vi "Tag initialize.vi"() -> (14 "RMS tag":refnum<class "NI Skyline Tag.lvclass">, 15 "RPM tag":refnum<class "NI Skyline Tag.lvclass">, 16 "Voltage tag":refnum<class "NI Skyline Tag.lvclass">, 17 "Current Tag":refnum<class "NI Skyline Tag.lvclass">, 18 "Temper tag":refnum<class "NI Skyline Tag.lvclass">, 19 "error out":errorcluster)   [LabVIEW 2017]
uses:
  <vilib>/Skyline/Tag/Wrapper/Wrapper_class/NI Skyline Tag.lvclass
  <vilib>/Skyline/Tag/Shared/typedefs/DataType.ctl
  <vilib>/Skyline/Tag/Wrapper/Wrapper AMQP_class/Open Tag AMQP.vi
  <vilib>/Skyline/Tag/Wrapper/Wrapper AMQP_class/NI Skyline Tag AMQP.lvclass
  <vilib>/Skyline/Tag/Shared/NI Skyline Tag.lvlib
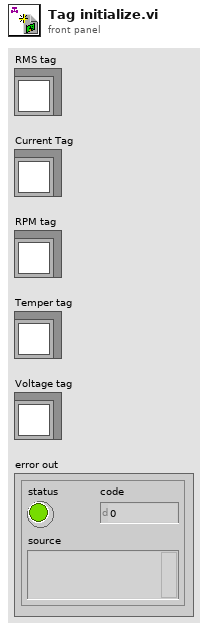
[diagram p1: front panel]
types:
  T1 = typedef "NI Skyline Tag.lvlib/DataType.ctl" = enum32{"Double", "I32", "String", "Boolean", "U64", "Timestamp"}
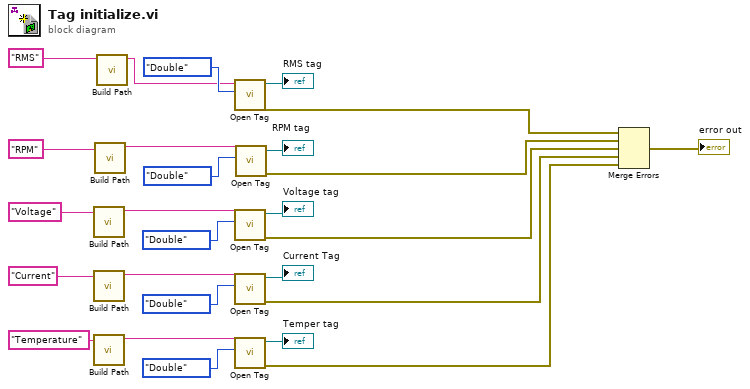
[diagram p0: block diagram]
diagram:
  n1 = call <vilib>:"Build Path.vi"("tag name"="Voltage" ("tag path")) -> ("path"=w9:string)  [unwired: 10 in]
  n2 = call <vilib>:"Build Path.vi"("tag name"="Current" ("tag path")) -> ("path"=w14:string)  [unwired: 10 in]
  n3 = call <vilib>:"Build Path.vi"("tag name"="Temperature" ("tag path")) -> ("path"=w15:string)  [unwired: 10 in]
  n4 = call <vilib>:"Build Path.vi"("tag name"="RPM" ("tag path")) -> ("path"=w7:string)  [unwired: 10 in]
  n5 = call <vilib>:"Build Path.vi"("tag name"="RMS" ("tag path")) -> ("path"=w5:string)  [unwired: 10 in]
  n6 = call-poly <vilib>:"Open Tag.vi"("data type"=DataType."Double" ("Data Type"), "path"=w5) -> ("error out"=w1:errorcluster, "tag out"=→"RMS tag":refnum<class "NI Skyline Tag.lvclass">)  [unwired: 8 in]
  n7 = call-poly <vilib>:"Open Tag.vi"("data type"=DataType."Double" ("Data Type"), "path"=w9) -> ("error out"=w18:errorcluster, "tag out"=→"Voltage tag":refnum<class "NI Skyline Tag.lvclass">)  [unwired: 8 in]
  n8 = call-poly <vilib>:"Open Tag.vi"("data type"=DataType."Double" ("Data Type"), "path"=w14) -> ("error out"=w19:errorcluster, "tag out"=→"Current Tag":refnum<class "NI Skyline Tag.lvclass">)  [unwired: 8 in]
  n9 = call-poly <vilib>:"Open Tag.vi"("data type"=DataType."Double" ("Data Type"), "path"=w15) -> ("error out"=w20:errorcluster, "tag out"=→"Temper tag":refnum<class "NI Skyline Tag.lvclass">)  [unwired: 8 in]
  n10 = call-poly <vilib>:"Open Tag.vi"("data type"=DataType."Double" ("Data Type"), "path"=w7) -> ("error out"=w2:errorcluster, "tag out"=→"RPM tag":refnum<class "NI Skyline Tag.lvclass">)  [unwired: 8 in]
  n11 = Merge Errors(w1, w2, w18, w19, w20) -> (→"error out":errorcluster)
